vi "DSF.Constants.vi"   [LabVIEW 2017, in "DSF Core.lvlib"]
uses:
  DSF Core.lvlib
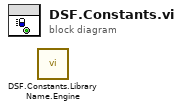
[diagram p0: block diagram]
diagram:
  n1 = call "DSF.Constants.Library Name.Engine.vi"() -> ()  [unwired: 11 in, 1 out]
